vi "TEST_bench_FXP_A_times_x_32bit.vi"(6 "NS":u8=9) -> ()   [LabVIEW 2017]
uses:
  fpga_subVIs_ssxy/fixed-point-ss/typeDefs/UT_matrix_data.ctl
  fpga_subVIs_ssxy/fixed-point-ss/typeDefs/Bz_vec_scalar.ctl
  fpga_subVIs_ssxy/fixed-point-ss/typeDefs/Lz_vec_scalar.ctl
  fpga_subVIs_ssxy/fixed-point-ss/typeDefs/Kz_vec_scalar.ctl
  fpga_subVIs_ssxy/fixed-point-ss/typeDefs/Nx_vec_scalar.ctl
  fpga_subVIs_ssxy/fixed-point-ss/typeDefs/Az_vec_scalar.ctl
  fpga_subVIs_ssxy/fixed-point-ss/typeDefs/x_vec_scalar.ctl
  fpga_subVIs_ssxy/fixed-point-ss/typeDefs/Cz_vec_scalar.ctl
  fpga_subVIs_ssxy/fixed-point-ss/typeDefs/x_vec_bram.ctl
  fpga_subVIs_ssxy/fixed-point-ss/typeDefs/A_as_vec_bram.ctl
  <vilib>/rvi/DataTransferAndStorage/Container/Common/niFpgaContainerExecOnDevCompGetState.vi
  <vilib>/rvi/Emulation/niFpgaEmulationIsFPGAContextNoSignature.vi
  <vilib>/rvi/DataTransferAndStorage/Container/Common/niFpgaContainerGetUniqueNameForEmu.vi
  <vilib>/rvi/Emulation/niFpgaProcessEmulError.vi
  <vilib>/rvi/Emulation/niFpgaSctlEmulationGetInTimedLoop.vi
  <vilib>/rvi/errors/nirviReportUnexpectedCaseInternalError (U32).vi
  <vilib>/rvi/Memory/Memory_Emulation/niFpgaMemoryEmulationCacheClearOnFirstRun.vi
  <vilib>/rvi/Memory/Memory_Emulation/nirvimemoryEmulationManagerCache_MakeExclusive.vi
  <vilib>/rvi/Memory/Memory_Emulation/niFpgaMemoryEmulationValidateCache.vi
  <vilib>/rvi/Memory/Memory_Emulation/nirvimemoryEmulationManagerCache_InsertValue.vi
  <vilib>/Utility/error.llb/Clear Errors.vi
  <vilib>/rvi/Memory/Memory_Emulation/nirvimemoryEmulationManagerCache_ReleaseExclusive.vi
  <vilib>/rvi/Memory/Memory_Emulation/nirvimemoryEmulationManagerCache_GetValue.vi
  <vilib>/rvi/Memory/Memory_Emulation/nirvimemoryEmulationManagerCache_SetValue.vi
  <vilib>/rvi/Emulation/niFpgaSctlEmulationResourceMgr.vi
  <vilib>/rvi/DataTransferAndStorage/Container/XNode/niFpgaContainer.xnode
  <vilib>/rvi/Memory/Memory_Emulation/niFpgaMemoryEmulationRefIn.vi
panel:
  in  "matrix data":T1
  out "xk_1_1":fxp<+/-,32,6>[](array[numeric])
  out "A*x":fxp<+/-,32,13>[](array[numeric])
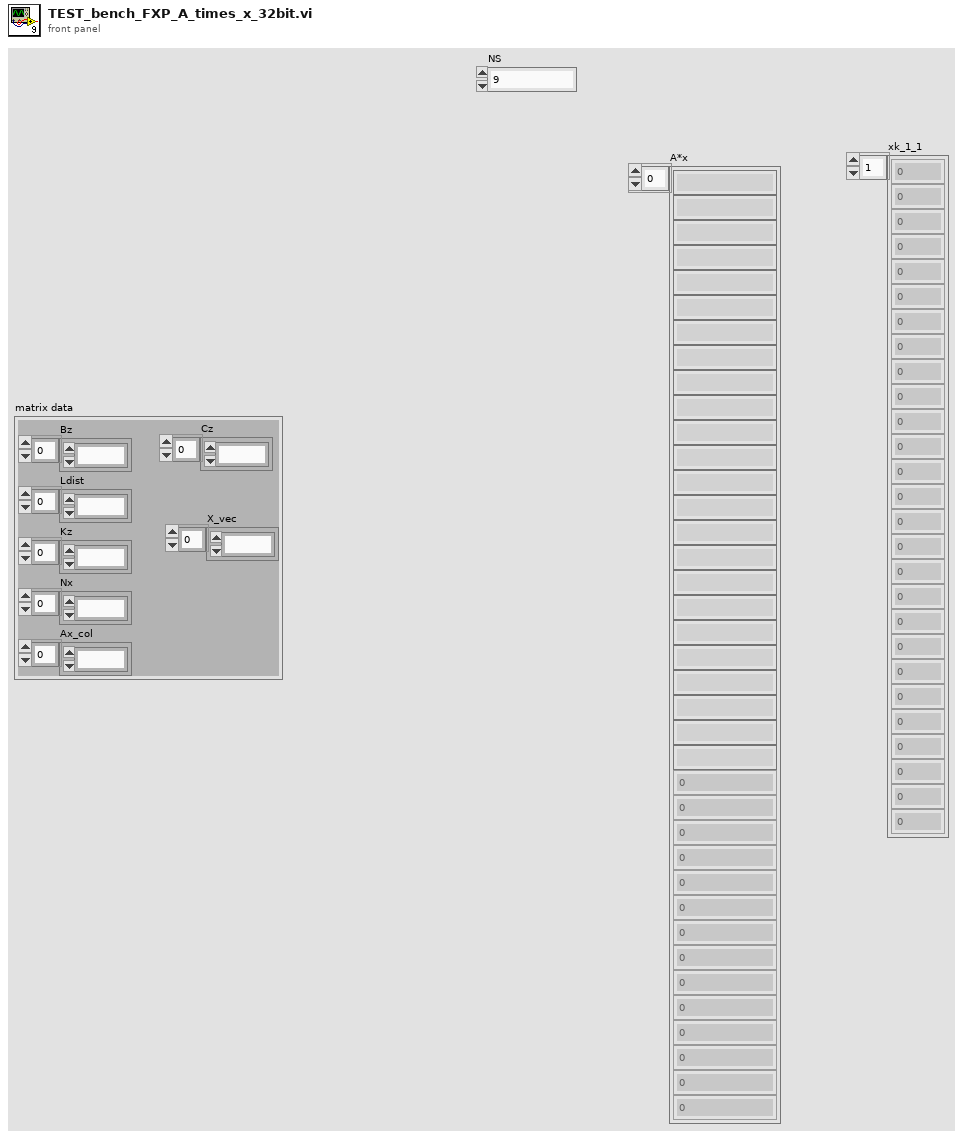
[diagram p1: front panel]
types:
  T1 = typedef "UT_matrix_data.ctl" = cluster{"Bz":T2[], "Ldist":T3[], "Kz":T4[], "Nx":T5[], "Ax_col":T6[], "X_vec":T7[], "Cz":T8[]}
  T2 = typedef "Bz_vec_scalar.ctl" = fxp<+/-,32,3>
  T3 = typedef "Lz_vec_scalar.ctl" = fxp<+/-,32,3>
  T4 = typedef "Kz_vec_scalar.ctl" = fxp<+/-,32,10>
  T5 = typedef "Nx_vec_scalar.ctl" = fxp<+/-,32,2>
  T6 = typedef "Az_vec_scalar.ctl" = fxp<+/-,32,7>
  T7 = typedef "x_vec_scalar.ctl" = fxp<+/-,32,6>
  T8 = typedef "Cz_vec_scalar.ctl" = fxp<+/-,32,4>
  T9 = typedef "x_vec_bram.ctl" = refnum<k21>
  T10 = typedef "A_as_vec_bram.ctl" = refnum<k21>
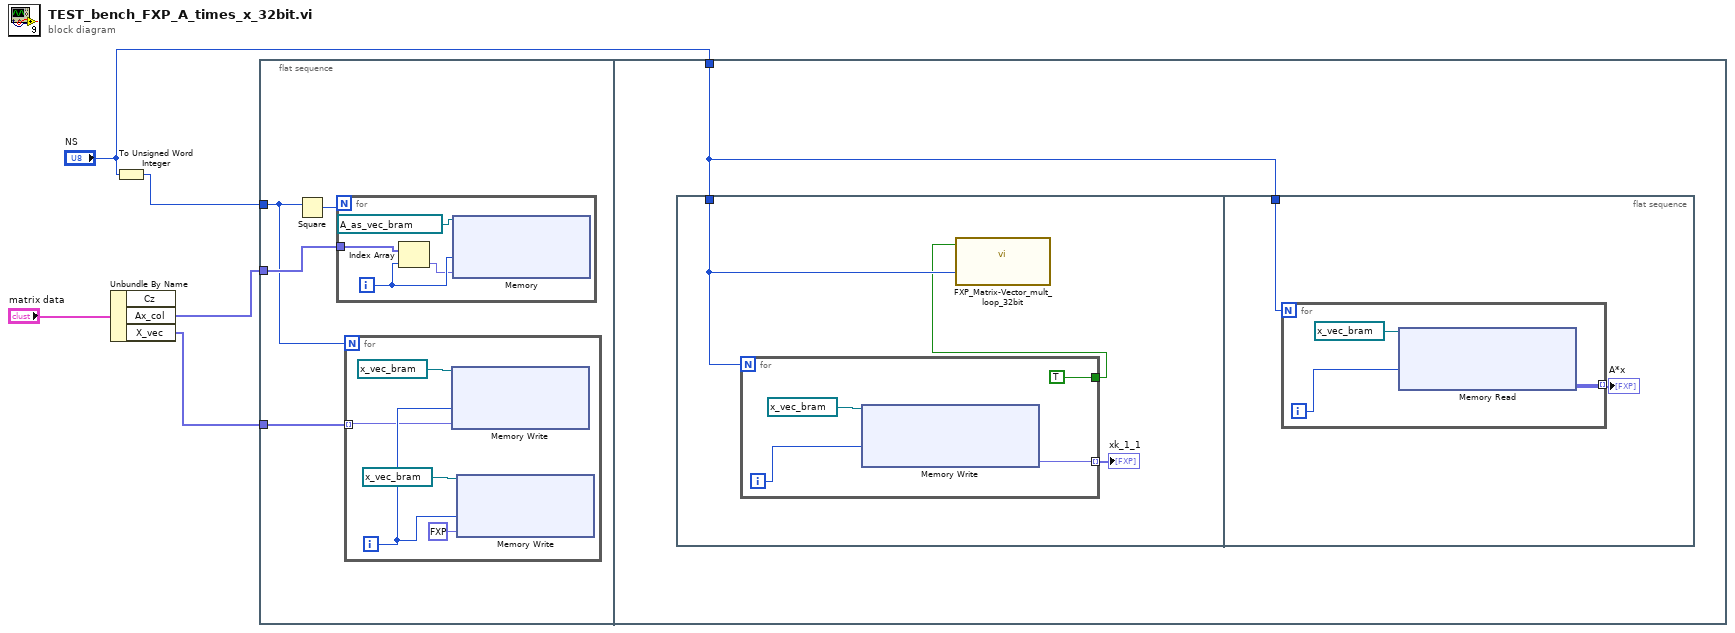
[diagram p0: block diagram]
diagram:
  n1 = Unbundle By Name("matrix data") -> ("Ax_col"=w5:T6[], "X_vec"=w4:T7[])  [unwired: 1 out]
  n2 = To Unsigned Word Integer(number="NS") -> (unsigned 16bit integer=w2:u16)
  n3 = flat-sequence {
    tunnel: w2 -> [w6]
    tunnel: w5 -> [w9]
    tunnel: w4 -> [w8]
    tunnel: "NS" -> [w19]
    frame #0 {
      n4 = Square(x=w6) -> (x^2=w7:u16)
      n5 = for {
        N: w7 -> [_]
        tunnel: w9 -> [w17]
        i -> [w16]
        n6 = Index Array(array=w17, index=w16) -> (element=w15:T6)
        n7 = xnode "Memory"("Address"=w16, "Data"=w15, "Memory In"=T10 "AasCol _FXP") -> ()  [unwired: 1 out]
      }
      n8 = for {
        N: w6 -> [_]
        tunnel: w8 -> [w11] mode=indexing
        i -> [w12]
        n9 = xnode "Memory Write"("Address"=w12, "Data"=w11, "Memory In"=T9 "xk_0_1" ("Memory")) -> ()  [unwired: 1 out]
        n10 = xnode "Memory Write"("Address"=w12, "Data"=fxp<+/-,32,6> 0.0, "Memory In"=T9 "xk_1_0" ("Memory")) -> ()  [unwired: 1 out]
      }
    }
    frame #1 {
      n11 = flat-sequence {
        tunnel: w19 -> [w22]
        tunnel: w19 -> [w27]
        frame #0 {
          n12 = for {
            N: w22 -> [_]
            tunnel: [w24] -> w21 mode=indexing
            tunnel: [TRUE] -> w20
            i -> [w25]
            n13 = xnode "Memory Write"("Address"=w25, "Memory In"=T9 "xk_0_1" ("Memory")) -> ("Data"=w24:fxp<+/-,32,6>)  [unwired: 1 out]
          }
          "xk_1_1" <- w21
          n14 = call "FXP_Matrix-Vector_mult_loop_32bit.vi"("Ns_1"=w22, "inputValid"=w20) -> ()  [unwired: 9 in, 1 out]
        }
        frame #1 {
          n15 = for {
            N: w27 -> [_]
            tunnel: [w30] -> w28 mode=indexing
            i -> [w29]
            n16 = xnode "Memory Read"("Address"=w29, "Memory In"=T9 "xk_1_0" ("Memory")) -> ("Data"=w30:fxp<+/-,32,6>)  [unwired: 1 out]
          }
          "A*x" <- w28
        }
      }
    }
  }
